vi "Order_Power_Spectrum_Processing.vi"(8 "element":T1, 11 "magnitude":dbl[](array[numeric])=[56.0, 155.5, 15.0]) -> (0 "Amplitudy rzêdów":dbl[](array[numeric]), 3 "sum":dbl)   [LabVIEW 2023]
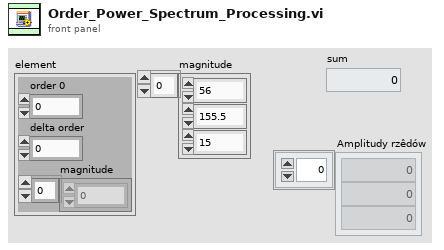
[diagram p1: front panel]
types:
  T1 = cluster{"order 0":dbl, "delta order":dbl, "magnitude":dbl[]}
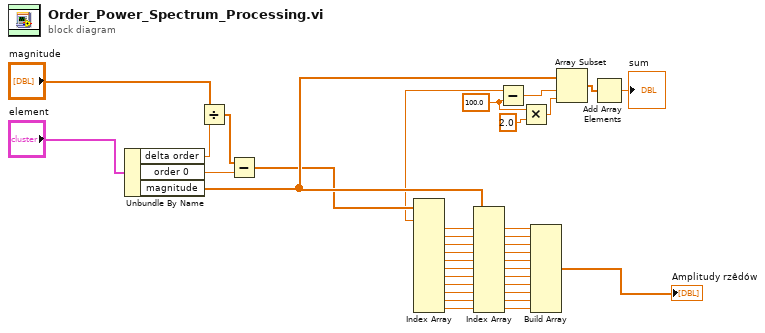
[diagram p0: block diagram]
diagram:
  w23 = 100.0 ("y")
  n1 = Unbundle By Name("element") -> ("delta order"=w36:dbl, "order 0"=w35:dbl, "magnitude"=w29:dbl[])
  n2 = Divide(x="magnitude", y=w36) -> (x/y=w37:dbl[])
  n3 = Subtract(x=w37, y=w35) -> (x-y=w22:dbl[])
  n4 = Index Array(array=w22) -> (element #1=w1:dbl, element #2=w21:dbl, element #3=w20:dbl, element #4=w19:dbl, element #5=w18:dbl, element #6=w17:dbl, element #7=w16:dbl, element #8=w15:dbl, element #9=w14:dbl, element #10=w13:dbl, element #11=w12:dbl, element #12=w4:dbl)  [unwired: 12 in]
  n5 = Index Array(array=w29, index #1=w21, index #2=w20, index #3=w19, index #4=w18, index #5=w17, index #6=w16, index #7=w15, index #8=w14, index #9=w13, index #10=w12, index #11=w4) -> (element #1=w33:dbl, element #2=w32:dbl, element #3=w31:dbl, element #4=w11:dbl, element #5=w10:dbl, element #6=w9:dbl, element #7=w8:dbl, element #8=w7:dbl, element #9=w6:dbl, element #10=w5:dbl, element #11=w3:dbl)
  n6 = Subtract(x=w1, y=w23) -> (x-y=w28:dbl)
  n7 = Multiply(x=w23, y=2.0) -> (x*y=w25:dbl)
  n8 = Build Array(w33, w32, w31, w11, w10, w9, w8, w7, w6, w5, w3) -> (→"Amplitudy rzêdów":dbl[])
  n9 = Array Subset(array=w29, index=w28, length=w25) -> (w27:dbl[])
  n10 = Add Array Elements(numeric array=w27) -> (sum=→"sum":dbl)
